vi "Y[i]=X[i-n] PtByPt (obs 90).vi"(2 "initialize":bool, 3 "shifts: n":i32, 5 "x":dbl format="%0.2f") -> (0 "error":i32, 1 "shifted x":dbl format="%0.2f")   [LabVIEW 2020, in "NI_PtbyPt.lvlib"]
uses:
  <vilib>/ptbypt/NI_PtbyPt.lvlib
panel:
  # "This VI is obsolete !!!\nYou should replace this VI in your diagram with the Y[i]=X[i-n] PtByPt VI.\n\nNOTE: Please be aware of that this obsolete VI shifts X[i-n+1] instead of\n            X[i-n]."
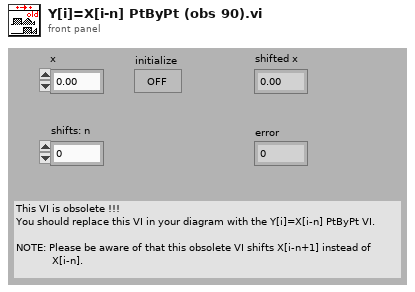
[diagram p1: front panel]
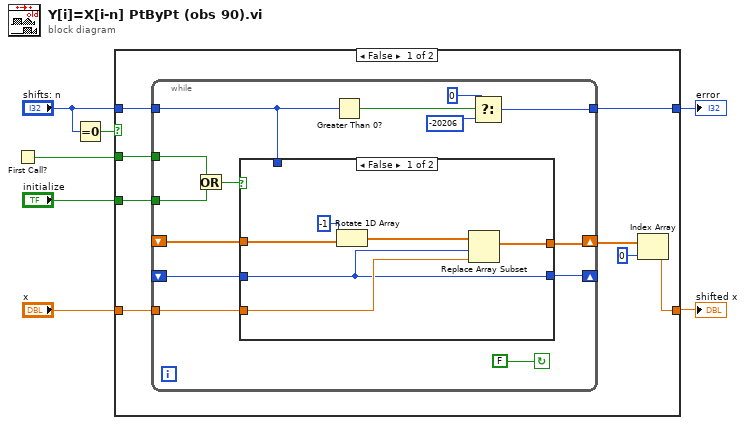
[diagram p0: block diagram]
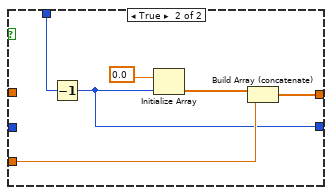
[diagram p2: hidden frame]
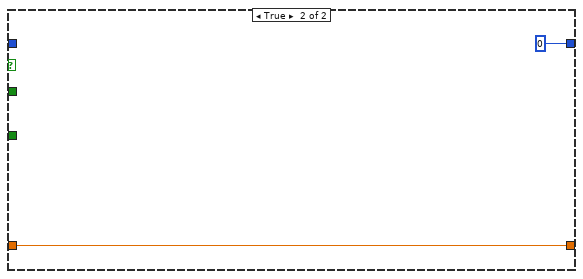
[diagram p3: hidden frame]
diagram:
  n1 = First Call?() -> (First Call?: T/F=w1:bool)
  n2 = Equal To 0?(x="shifts: n") -> (x = 0?=w3:bool)
  n3 = case shown="False" w3 {
    tunnel: "x" -> [w13 w42]
    tunnel: [w8 w42] -> w6
    tunnel: [w11 0 ("error")] -> w5
    tunnel: "shifts: n" -> [w12 _]
    tunnel: "initialize" -> [w15 _]
    tunnel: w1 -> [w14 _]
    frame False {
      n4 = while {
        tunnel: [w16] -> w11
        tunnel: w12 -> [w17]
        tunnel: w13 -> [w21]
        tunnel: w14 -> [w22]
        tunnel: w15 -> [w23]
        shift-left: _ -> [w27]
        shift-right: [w28] -> _
        shift-left: _ -> [w26]
        shift-right: [w29] -> w9
        stop <- FALSE continue-if-true
        n5 = Or(x=w22, y=w23) -> (x .or. y?=w24:bool)
        n6 = case shown="False" w24 {
          tunnel: [w33 w39] -> w29
          tunnel: [w30 w36] -> w28
          tunnel: w27 -> [w30 _]
          tunnel: w26 -> [w31 _]
          tunnel: w21 -> [w34 w41]
          tunnel: w17 -> [_ w37]
          frame False {
            n7 = Rotate 1D Array(1:w31, 2:i16 -1 ("n")) -> (0:w32:dbl[])
            n8 = Replace Array Subset(array=w32, new element=w34, index=w30) -> (w33:dbl[])
          }
          frame True {
            n9 = Decrement(x=w37) -> (x-1=w36:i32)
            n10 = Initialize Array(0.0 ("Element Data"), w36) -> (w38:dbl[])
            n11 = Build Array (concatenate)(w38, w41) -> (w39:dbl[])
          }
        }
        n12 = Greater Than 0?(x=w17) -> (x > 0?=w18:bool)
        n13 = Select(t=0, s=w18, f=-20206) -> (s? t:f=w16:i32)
      }
      n14 = Index Array(array=w9, index=0 ("Index")) -> (element=w8:dbl)
    }
    frame True {
    }
  }
  "shifted x" <- w6
  "error" <- w5
